vi "Write Timestamp.vi"(10 "Timestamp":timestamp, 11 "Timestamp Event in":refnum<class "Timestamp Event.lvclass">) -> (3 "Timestamp Event out":refnum<class "Timestamp Event.lvclass">)   [LabVIEW 2016, in "Example Source.lvlib" / "Timestamp Event.lvclass"]
uses:
  Timestamp Event.lvclass
  Timestamp Event.lvclass/Timestamp Event.ctl
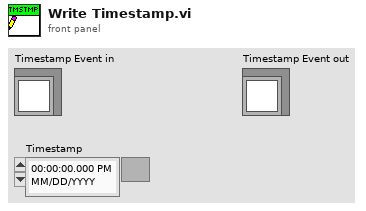
[diagram p1: front panel]
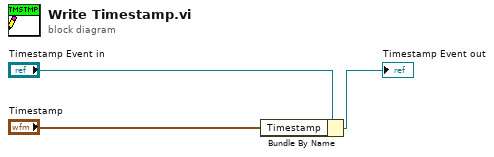
[diagram p0: block diagram]
diagram:
  n1 = Bundle By Name(cluster="Timestamp Event in", "Timestamp"="Timestamp") -> (→"Timestamp Event out":refnum<class "Timestamp Event.lvclass">)
